vi "Teleop.vi"   [LabVIEW 2016]
doc: "This VI is called for each TeleOp packet received from the DS where the robot is not disabled. It is often used to read from the joysticks and update I/O or to update setpoints for timed control loops. It should complete and return within 20 milliseconds or it may miss DS packets."
uses:
  <vilib>/Rock Robotics/WPI/Utilities/WPI_GetSetVariantRefNum.vi
  External/2ndContollerStatus.vi
  External/External.lvlib
types:
  T1 = enum16{"A", "B", "X", "Y", "LB", "RB", "Back", "Start", "Left Joystick Pressure Button", "Right Joystick Pressure Button"}
  T2 = enum16{"Left X Axis", "Left Y Axis", "Left Trigger", "Right Trigger", "Right X Axis", "Right Y Axis"}
  T3 = typedef "WPI_JoystickDevRef.ctl" = cluster{"Device":T4}
  T4 = typedef "WPI_JoystickDeviceEnum.ctl" = enum16{"USB 0", "USB 1", "USB 2", "USB 3", "USB 4", "USB 5"}
  T5 = typedef "WPI_RobotDriveDevRef.ctl" = cluster{"DevStatus":errorcluster, "Motors[]":T6[], "Square Inputs":bool, "Max Output":dbl}
  T6 = typedef "WPI_MotorControlDeviceRef.ctl" = cluster{"DeviceStatus":errorcluster, "Type":T7, "PWM":cluster{"PWM Channel":T8, "DeadBand":T9}, "CAN":cluster{"Device Number":u8, "SetOutput VI Ref":variant, "GetOutput VI Ref":variant, "Enable VI Ref":variant, "Disable VI Ref":variant, "Data":variant}, "Invert":bool}
  T7 = typedef "WPI_MotorControlType.ctl" = enum16{"PWM", "CAN"}
  T8 = typedef "FPGA_DIOPWMChannel.ctl" = enum8{"PWM 0", "PWM 1", "PWM 2", "PWM 3", "PWM 4", "PWM 5", "PWM 6", "PWM 7", "PWM 8", "PWM 9", "PWM MXP 0", "PWM MXP 1", "PWM MXP 2", "PWM MXP 3", "PWM MXP 4", "PWM MXP 5", "PWM MXP 6", "PWM MXP 7", "PWM MXP 8", "PWM MXP 9", "Invalid"}
  T9 = typedef "WPI_PWMDeadband.ctl" = cluster{"Name":string, "maxPositivePwm":i32, "minPositivePwm":i32, "centerPwm":i32, "maxNegativePwm":i32, "minNegativePwm":i32, "angularRange":u16}
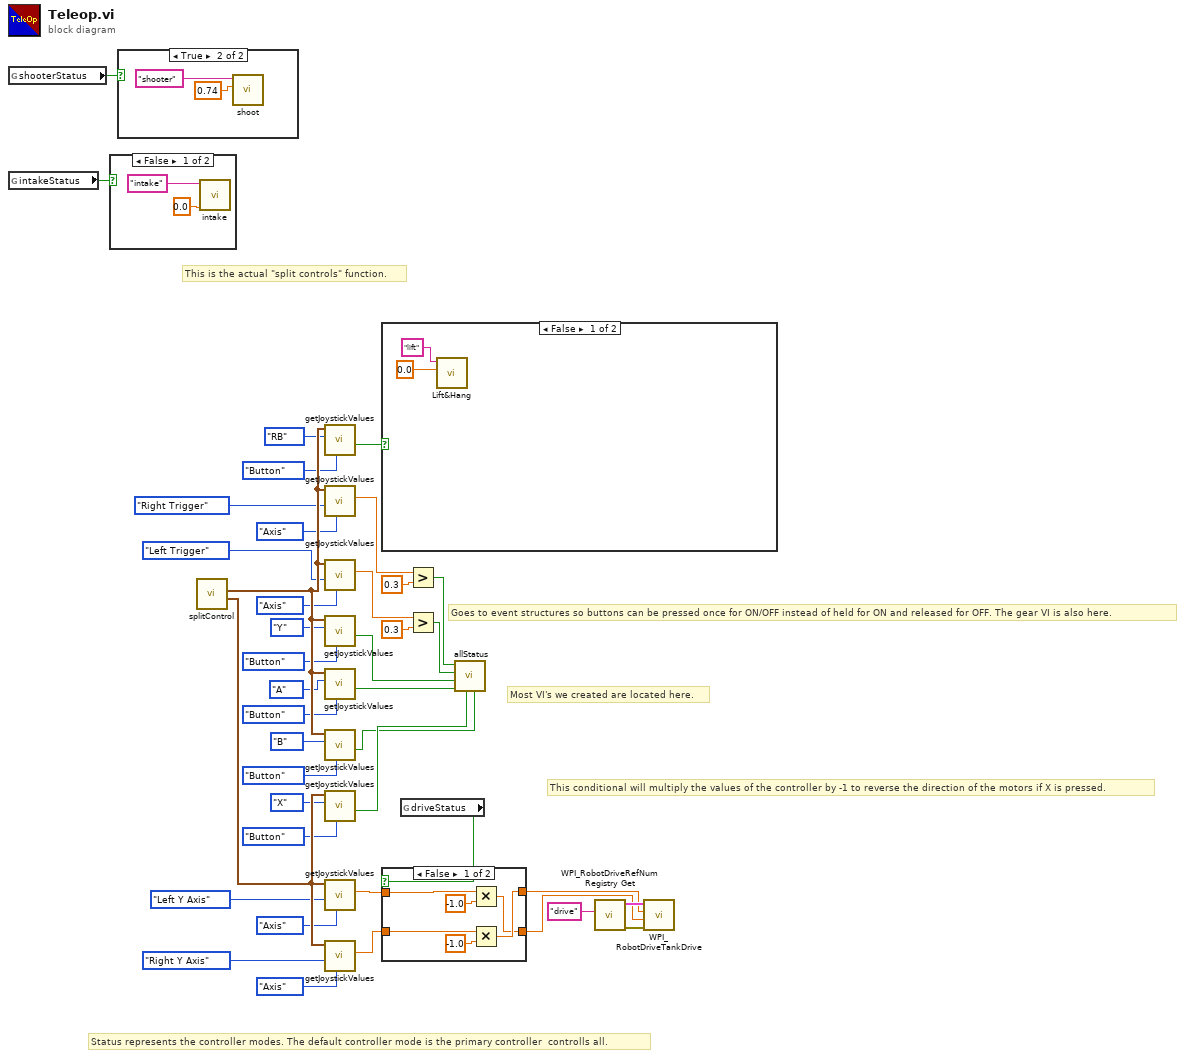
[diagram p0: block diagram]
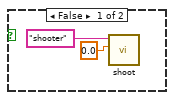
[diagram p3: hidden frame]
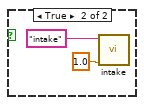
[diagram p4: hidden frame]
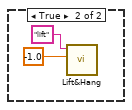
[diagram p5: hidden frame]
diagram:
  # "This is the actual \"split controls\" function."
  # "Most VI's we created are located here."
  # "This conditional will multiply the values of the controller by -1 to reverse the direction of the motors if X is pressed."
  # "Goes to event structures so buttons can be pressed once for ON/OFF instead of held for ON and released for OFF. The gear VI is also here."
  # "Status represents the controller modes. The default controller mode is the primary controller  controlls all."
  n1 = global read "2ndContollerStatus.vi" "shooterStatus"() -> (w32:bool)
  n2 = global read "2ndContollerStatus.vi" "intakeStatus"() -> (w33:bool)
  n3 = case shown="False" w33 {
    frame False {
      n4 = call "intake.vi"("intakeSpeed"=0.0, "intake"="intake") -> ()  [unwired: 9 in, 1 out]
    }
    frame True {
      n5 = call "intake.vi"("intakeSpeed"=1.0, "intake"="intake") -> ()  [unwired: 9 in, 1 out]
    }
  }
  n6 = case shown="True" w32 {
    frame False {
      n7 = call "shoot.vi"("Motor Power"=0.0, "refnum name"="shooter") -> ()  [unwired: 9 in, 1 out]
    }
    frame True {
      n8 = call "shoot.vi"("Motor Power"=0.74, "refnum name"="shooter") -> ()  [unwired: 9 in, 1 out]
    }
  }
  n9 = call "splitControl.vi"() -> ("JoystickDevRef 2"=w20:T3, "JoystickDevRef"=w21:T3)  [unwired: 10 in]
  n10 = call "getJoystickValues.vi"("Mode"=enum16{"Axis", "Button", "POV"}."Button", "buttonType"=T1."RB", "JoystickDevRef"=w21) -> ("Button Pressed"=w41:bool)  [unwired: 5 in, 3 out]
  n11 = call "getJoystickValues.vi"("Mode"=enum16{"Axis", "Button", "POV"}."Axis", "axisType"=T2."Right Trigger", "JoystickDevRef"=w21) -> ("Value"=w35:dbl)  [unwired: 5 in, 3 out]
  n12 = call "getJoystickValues.vi"("Mode"=enum16{"Axis", "Button", "POV"}."Axis", "axisType"=T2."Left Trigger", "JoystickDevRef"=w21) -> ("Value"=w34:dbl)  [unwired: 5 in, 3 out]
  n13 = call "getJoystickValues.vi"("Mode"=enum16{"Axis", "Button", "POV"}."Button", "buttonType"=T1."Y", "JoystickDevRef"=w21) -> ("Button Pressed"=w19:bool)  [unwired: 5 in, 3 out]
  n14 = call "getJoystickValues.vi"("Mode"=enum16{"Axis", "Button", "POV"}."Button", "buttonType"=T1."A", "JoystickDevRef"=w21) -> ("Button Pressed"=w24:bool)  [unwired: 5 in, 3 out]
  n15 = call "getJoystickValues.vi"("Mode"=enum16{"Axis", "Button", "POV"}."Button", "buttonType"=T1."B", "JoystickDevRef"=w21) -> ("Button Pressed"=w22:bool)  [unwired: 5 in, 3 out]
  n16 = call "getJoystickValues.vi"("Mode"=enum16{"Axis", "Button", "POV"}."Button", "buttonType"=T1."X", "JoystickDevRef"=w20) -> ("Button Pressed"=w23:bool)  [unwired: 5 in, 3 out]
  n17 = call "getJoystickValues.vi"("Mode"=enum16{"Axis", "Button", "POV"}."Axis", "axisType"=T2."Left Y Axis", "JoystickDevRef"=w20) -> ("Value"=w30:dbl)  [unwired: 5 in, 3 out]
  n18 = call "getJoystickValues.vi"("Mode"=enum16{"Axis", "Button", "POV"}."Axis", "axisType"=T2."Right Y Axis", "JoystickDevRef"=w20) -> ("Value"=w28:dbl)  [unwired: 5 in, 3 out]
  n19 = case shown="False" w41 {
    frame False {
      n20 = call "Lift&Hang.vi"("status"=0.0, "refnum name"="lift" ("lift")) -> ()  [unwired: 9 in, 1 out]
    }
    frame True {
      n21 = call "Lift&Hang.vi"("status"=-1.0, "refnum name"="lift" ("lift")) -> ()  [unwired: 9 in, 1 out]
    }
  }
  n22 = global read "2ndContollerStatus.vi" "driveStatus"() -> (w27:bool)
  n23 = case shown="False" w27 {
    tunnel: [w55 w61] -> w31
    tunnel: w30 -> [w59 w61]
    tunnel: [w54 w60] -> w29
    tunnel: w28 -> [w57 w60]
    frame False {
      n24 = Multiply(x=w59, y=-1.0) -> (x*y=w54:dbl)
      n25 = Multiply(x=w57, y=-1.0) -> (x*y=w55:dbl)
    }
    frame True {
    }
  }
  n26 = Greater?(x=w35, y=0.3) -> (0:w26:bool)
  n27 = Greater?(x=w34, y=0.3) -> (0:w25:bool)
  n28 = call "allStatus.vi"("intake"=w22, "drive"=w23, "gear"=w24, "shooter"=w19, "hopper1"=w25, "hopper0"=w26) -> ()  [unwired: 6 in]
  n29 = call <vilib>:"WPI_RobotDriveRefNum Registry Get.vi"("refnum name"="drive") -> ("error out"=w39:errorcluster, "RobotDriveDevRef"=w40:T5)  [unwired: 9 in]
  n30 = call <vilib>:"WPI_RobotDriveTankDrive.vi"("error in (no error)"=w39, "Right axis value"=w29, "Left axis value"=w31, "RobotDriveDevRef"=w40) -> ()  [unwired: 5 in, 3 out]
